vi "NoAndStatus.vi"(5 "experiment_no":i32, 7 "vial_no":i32, 8 "error in (no error)":errorcluster, 9 "Python version":string, 11 "user.xls path":path) -> (0 "error out":errorcluster)   [LabVIEW 2020]
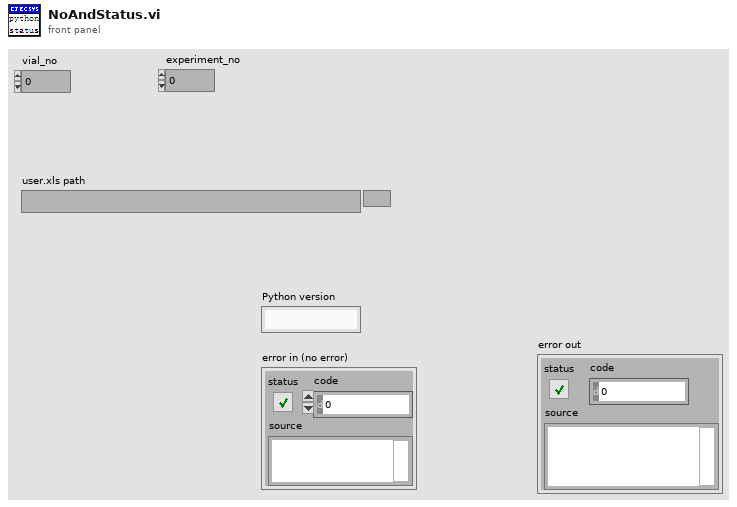
[diagram p1: front panel]
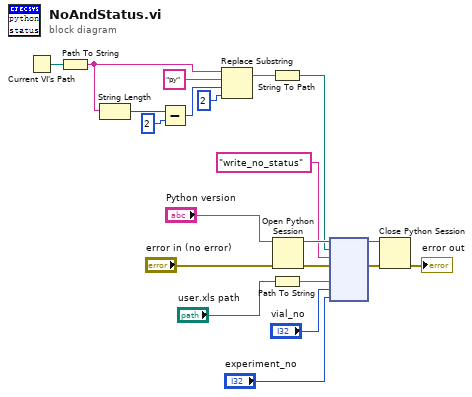
[diagram p0: block diagram]
diagram:
  n1 = Current VI's Path() -> (path=w11:path)
  n2 = Path To String(path=w11) -> (string=w10:string)
  n3 = String Length(string=w10) -> (length=w7:i32)
  n4 = Subtract(x=w7, y=2) -> (x-y=w6:i32)
  n5 = Replace Substring(2:2 ("length (len. of substring)"), 3:w6, 4:"py" ("substring (\"\")"), 5:w10) -> (1:w4:string)  [unwired: 1 out]
  n6 = String To Path(string=w4) -> (path=w3:path)
  n7 = Path To String(path="user.xls path") -> (string=w13:string)
  n8 = Open Python Session(python version="Python version", 3:"error in (no error)") -> (session out=w20:refnum<k35>, error out=w17:errorcluster)  [unwired: 1 in]
  n9 = node(w20, w3, "write_no_status" ("function name"), w17, w13, "vial_no", "experiment_no") -> (w19:refnum<k35>, w18:errorcluster)  [unwired: 5 in, 2 out]
  n10 = Close Python Session(session in=w19, error in=w18) -> (11:→"error out":errorcluster)
